vi "3446X_Close.vi"(0 "User Reference":i32, 5 "error in (no error)":errorcluster) -> (19 "error out":errorcluster)   [LabVIEW 2015, in "3446X.lvclass"]
uses:
  3446X.lvclass
  DMM Virtual/DMM Virtual.lvclass
  <instrlib>/Agilent 3446X Series/Agilent 3446X Series.lvlib
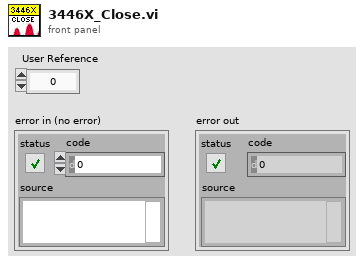
[diagram p1: front panel]
types:
  T1 = typedef "Class Attributes Cluster.ctl" = cluster{"Model Number":string, "Instrument Number":u8, "Rack ID":string, "Inst Mnemonic":string, "Comp Mnemonic":string, "Subsys Mnemonic":string, "IP Address":string, "Sub Address":string, "Firmware Rev":string, "Expected Options":string, "Required Options":string, "Excluded Options":string}
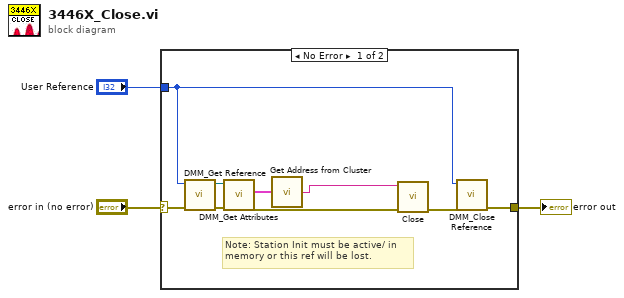
[diagram p0: block diagram]
diagram:
  n1 = case shown="No Error" "error in (no error)" {
    selector: "error in (no error)" -> [w12 w13]
    tunnel: [w8 w13] -> w2
    tunnel: "User Reference" -> [w11 _]
    frame No Error {
      # "Note: Station Init must be active/ in\nmemory or this ref will be lost."
      n2 = call "DMM_Get Reference.vi"("error in (no error)"=w12, "Instrument Reference"=w11) -> ("error out"=w9:errorcluster, "DMM Virtual.lvclass"=w10:refnum<class "DMM Virtual.lvclass">)  [unwired: 8 in]
      n3 = call-dynamic "DMM_Get Attributes.vi"("error in (no error)"=w9, "DMM Virtual in"=w10) -> ("error out"=w7:errorcluster, "Class Attributes"=w5:T1)  [unwired: 7 in, 1 out]
      n4 = call "Get Address from Cluster.vi"("Class Attributes"=w5) -> ("Address"=w4:string)  [unwired: 4 in]
      n5 = call <instrlib>:"Close.vi"("error in (no error)"=w7, "VISA resource name"=w4) -> ("error out"=w6:errorcluster)  [unwired: 9 in]
      n6 = call "DMM_Close Reference.vi"("error in (no error)"=w6, "User Reference"=w11) -> ("error out"=w8:errorcluster)  [unwired: 9 in]
    }
    frame Error {
    }
  }
  "error out" <- w2
